vi "Endpoint Aliases Page.vi"(8 "error in (no error)":errorcluster, 11 "Node Ptr":T5 format="%.0x") -> (0 "error out":errorcluster)   [LabVIEW 2017, in "Routing and Faulting System Explorer.lvlib"]
uses:
  Routing and Faulting System Explorer.lvlib
  <vilib>/NI Veristand/Custom Device API/Custom Device Item Ref.ctl
  Alias.ctl
  Endpoint.ctl
  Shared/UI Common/Sort Button.ctl
  Shared/UI Common/Add Button.ctl
  Aliases Page Controls.ctl
  9b1be06d-3bcf-4b89-8ea1-6f7bb6167b61.vi
  Shared/UI Common/Set Control Value.vi
  <vilib>/NI Veristand/Custom Device API/Custom Device API.lvlib
  Shared/UI Common/UI Common.lvlib
  Scripting/Routing and Faulting Scripting.lvlib
panel:
  in  "Items to add":dbl=5.0
  in  "Add Alias":T1
  in  "Sort":T2
  out "Alias":string="Alias"
  out "Endpoint":string="Endpoint"
  in  "Aliases":T3[](array[typedef])
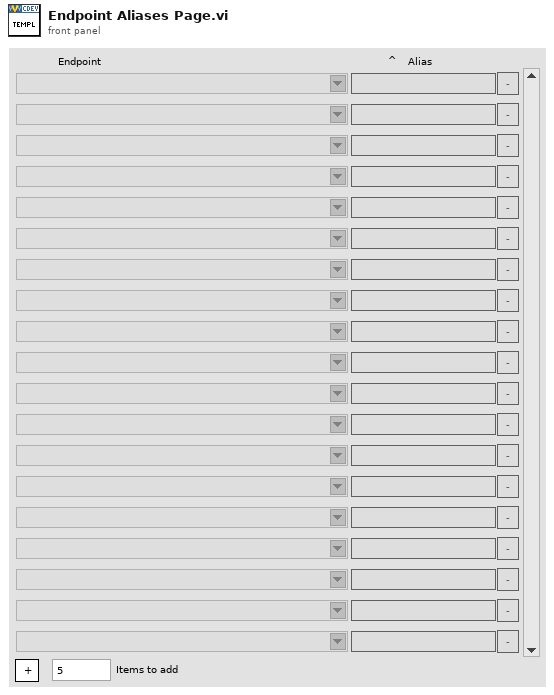
[diagram p1: front panel]
types:
  T1 = typedef "UI Common.lvlib/Add Button.ctl" = bool
  T2 = typedef "UI Common.lvlib/Sort Button.ctl" = bool
  T3 = typedef "Routing and Faulting System Explorer.lvlib/Alias.ctl" = cluster{"Endpoint":T4, "Alias":string, "Remove":bool}
  T4 = typedef "Routing and Faulting System Explorer.lvlib/Endpoint.ctl" = string
  T5 = typedef "Custom Device API.lvlib/Custom Device Item Ref.ctl" = u64
  T6 = typedef "Routing and Faulting System Explorer.lvlib/Aliases Page Controls.ctl" = cluster{"Aliases":refnum<vi>, "Endpoint":refnum<vi>, "Alias":refnum<vi>, "Sort":refnum<vi>}
  T7 = typedef "Custom Device API.lvlib/Custom Device Commands.ctl" = enum16{"Default", "Item renamed", "Shutdown", "Dynamic button pressed"}
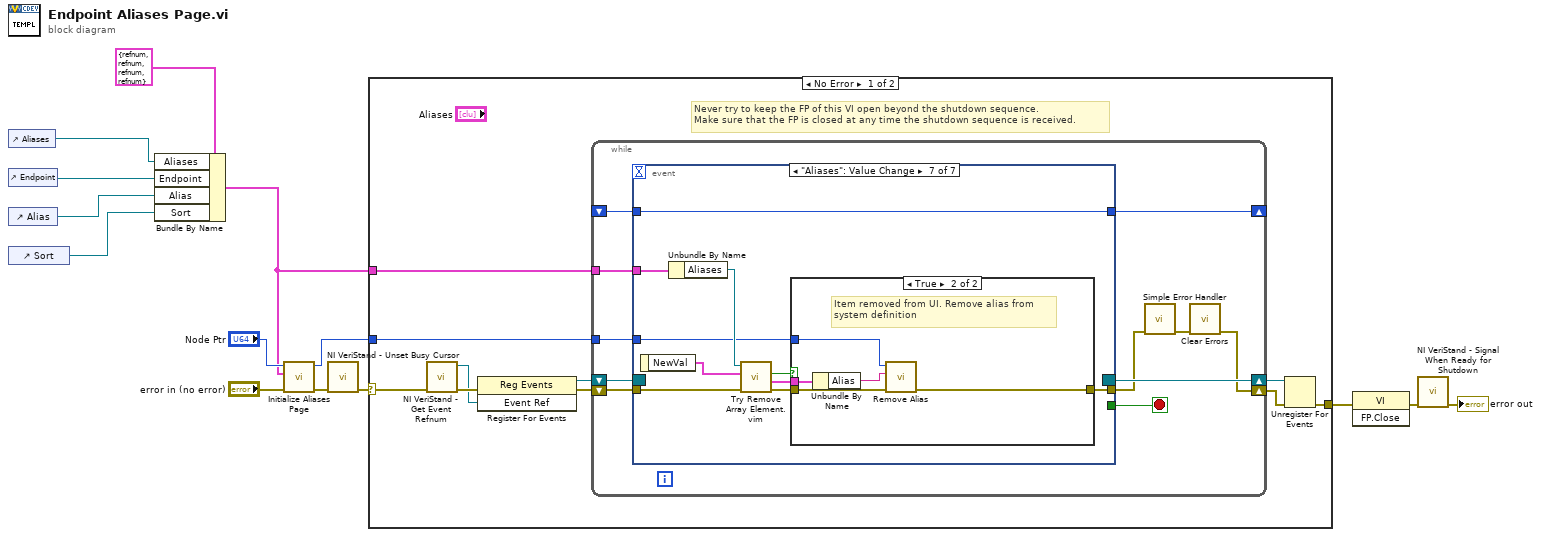
[diagram p0: block diagram]
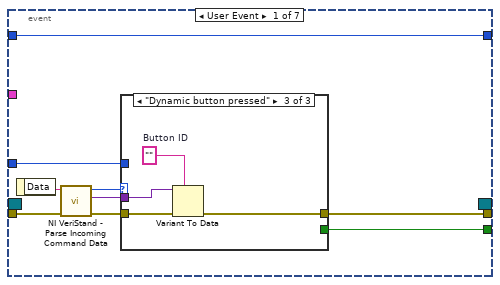
[diagram p2: hidden frame]
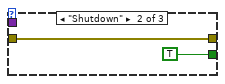
[diagram p4: hidden frame]
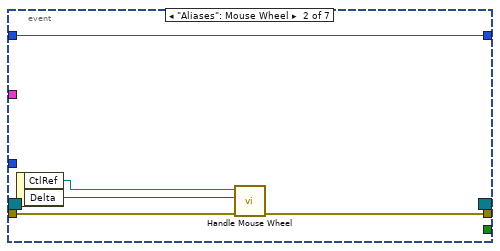
[diagram p5: hidden frame]
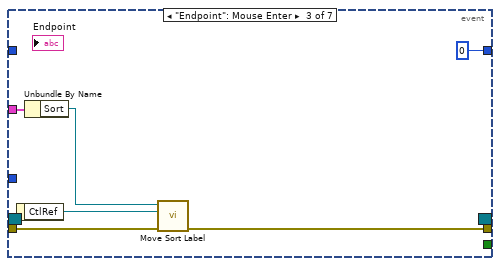
[diagram p6: hidden frame]
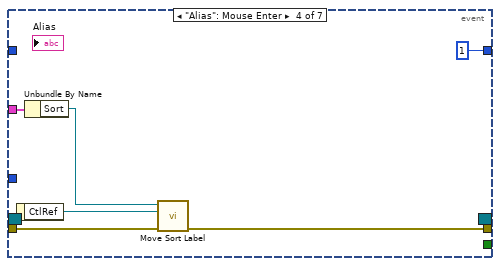
[diagram p7: hidden frame]
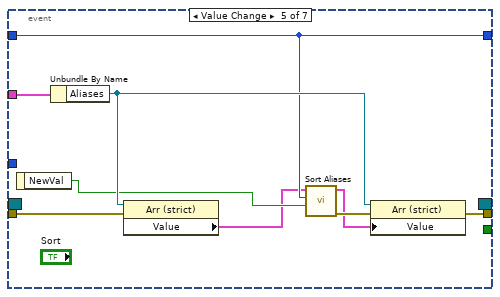
[diagram p8: hidden frame]
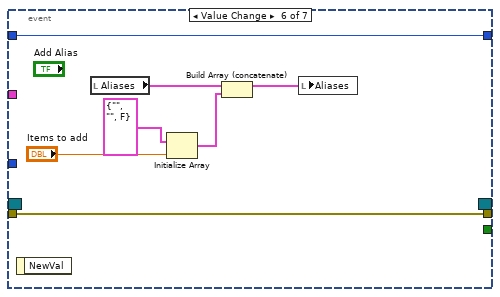
[diagram p9: hidden frame]
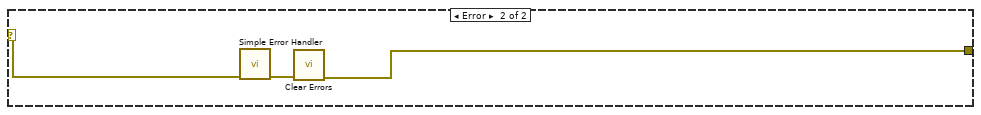
[diagram p11: hidden frame]
diagram:
  n1 = control-ref of="Aliases"() -> (w1:refnum<vi>)
  n2 = control-ref of="Endpoint"() -> (w8:refnum<vi>)
  n3 = control-ref of="Alias"() -> (w7:refnum<vi>)
  n4 = control-ref of="Sort"() -> (w6:refnum<vi>)
  n5 = Bundle By Name(cluster=T6 {"Aliases"=refnum, "Endpoint"=refnum, "Alias"=refnum, "Sort"=refnum} ("Aliases Page Controls"), "Aliases"=w1, "Endpoint"=w8, "Alias"=w7, "Sort"=w6) -> (w2:T6)
  n6 = call "Initialize Aliases Page.vi"("error in (no error)"="error in (no error)", "Aliases Page Controls"=w2, "Aliases Ref in"="Node Ptr") -> ("error out"=w5:errorcluster, "Aliases Ref out"=w9:T5)  [unwired: 7 in]
  n7 = call <vilib>:"NI VeriStand - Unset Busy Cursor.vi"("error in (no error)"=w5) -> ("error out"=w12:errorcluster)  [unwired: 10 out]
  n8 = case shown="No Error" w12 {
    selector: w12 -> [w19 w103]
    tunnel: [w22 w101] -> w14
    tunnel: w9 -> [w20 _]
    tunnel: w2 -> [w17 _]
    frame No Error {
      # "Never try to keep the FP of this VI open beyond the shutdown sequence.\nMake sure that the FP is closed at any time the shutdown sequence is received."
      n9 = call <vilib>:"NI VeriStand - Get Event Refnum.vi"("error in (no error)"=w19) -> ("error out"=w16:errorcluster, "Event Ref"=w15:refnum<user-event>)  [unwired: 9 out]
      n10 = register-events(error in=w16, w15) -> (reference out=w21:refnum<event-registration>, error out=w18:errorcluster)  [unwired: 1 in]
      n11 = while {
        tunnel: w20 -> [w31]
        shift-right: [w28] -> w23
        shift-left: w18 -> [w34]
        shift-right: [w35] -> w24
        shift-left: w21 -> [w33]
        shift-right: [w27] -> _
        shift-left: _ -> [w25]
        tunnel: w17 -> [w26]
        stop <- w32 stop-if-true
        n12 = event shown="[6] \"Aliases\": Value Change" {
          selector: w33 -> [_ _ _ _ _ _ _]
          dyn-events: [_ _ _ _ _ _ _] -> w35
          timeout: _ -> [_ _ _ _ _ _ _]
          tunnel: w34 -> [w44 w54 w62 w68 w77 w82 w93]
          tunnel: [w40 _ _ _ _ _ _] -> w32
          tunnel: [w39 w53 w61 w67 w74 w82 w87] -> w30
          tunnel: w31 -> [w38 _ _ _ _ _ w85]
          tunnel: [w36 w56 0 ("index of element") 1 ("index of element") w71 w84 w94] -> w27
          tunnel: w26 -> [_ _ w58 w64 w76 _ w91]
          tunnel: w25 -> [w36 w56 _ _ w71 w84 w94]
          event User Event {
            n13 = event-data() -> ("Data"=w43:string)  [unwired: 1 out]
            n14 = call <vilib>:"NI VeriStand - Parse Incoming Command Data.vi"("error in (no error)"=w44, "Incoming data"=w43) -> ("error out"=w42:errorcluster, "Outgoing data"=w37:variant, "Action"=w41:T7)  [unwired: 7 out]
            n15 = case shown="\"Dynamic button pressed\"" w41 {
              tunnel: w42 -> [w45 w46 w51]
              tunnel: [_ TRUE _] -> w40
              tunnel: [w45 w46 w48] -> w39
              tunnel: w38 -> [_ _ _]
              tunnel: w37 -> [_ _ w50]
              frame "Default", Default {
              }
              frame "Shutdown" {
              }
              frame "Dynamic button pressed" {
                w49 = ""  # Button ID
                n16 = Variant To Data(error in=w51, type=w49, Variant=w50) -> (error out=w48:errorcluster)  [unwired: 1 out]
              }
            }
          }
          event "Aliases": Mouse Wheel {
            n17 = event-data() -> ("CtlRef"=w55:refnum<vi>, "Delta"=w52:i32)  [unwired: 1 out]
            n18 = call "Handle Mouse Wheel.vi"("error in (no error)"=w54, "delta"=w52, "Array Refnum"=w55) -> ("error out"=w53:errorcluster)  [unwired: 7 in, 1 out]
          }
          event "Endpoint": Mouse Enter {
            n19 = event-data() -> ("CtlRef"=w60:refnum<vi>)  [unwired: 1 out]
            n20 = Unbundle By Name(w58) -> ("Sort"=w57:refnum<vi>)
            n21 = call "Move Sort Label.vi"("error in (no error)"=w62, "Target Label"=w60, "Sort"=w57) -> ("error out"=w61:errorcluster)  [unwired: 8 in]
          }
          event "Alias": Mouse Enter {
            n22 = event-data() -> ("CtlRef"=w66:refnum<vi>)  [unwired: 1 out]
            n23 = Unbundle By Name(w64) -> ("Sort"=w63:refnum<vi>)
            n24 = call "Move Sort Label.vi"("error in (no error)"=w68, "Target Label"=w66, "Sort"=w63) -> ("error out"=w67:errorcluster)  [unwired: 8 in]
          }
          event Value Change {
            n25 = event-data() -> ("NewVal"=w72:T2)  [unwired: 1 out]
            n26 = Unbundle By Name(w76) -> ("Aliases"=w73:refnum<vi>)
            n27 = property class="Arr (strict)"(reference=w73, error in=w77) -> ("Value"=w69:T3[])  [unwired: 2 out]
            n28 = call "Sort Aliases.vi"("Descending"=w72, "index"=w71, "Aliases"=w69) -> ("error out"=w75:errorcluster, "Sorted Aliases"=w70:T3[])  [unwired: 7 in]
            n29 = property class="Arr (strict)"(reference=w73, error in=w75, "Value"=w70) -> (error out=w74:errorcluster)  [unwired: 1 out]
          }
          event Value Change {
            n30 = event-data() -> ()  [unwired: 2 out]
            n31 = local read "Aliases"() -> (w80:T3[])
            n32 = Initialize Array(T3 {"Endpoint"="", "Alias"="", "Remove"=FALSE} ("Alias"), "Items to add") -> (w79:T3[])
            n33 = Build Array (concatenate)(w80, w79) -> (w78:T3[])
            n34 = local write "Aliases"(w78) -> ()
          }
          event "Aliases": Value Change {
            n35 = event-data() -> ("NewVal"=w92:T3[])  [unwired: 1 out]
            n36 = Unbundle By Name(w91) -> ("Aliases"=w90:refnum<vi>)
            n37 = call "Try Remove Array Element.vim"("error in (no error)"=w93, "Array"=w92, "Ctl Refnum"=w90) -> ("error out"=w88:errorcluster, "Removed Item"=w86:T3, "Removed?"=w89:bool)  [unwired: 5 in, 1 out]
            n38 = case shown="True" w89 {
              tunnel: w88 -> [w95 w99]
              tunnel: [w95 w98] -> w87
              tunnel: w86 -> [_ w100]
              tunnel: w85 -> [_ w96]
              frame False {
                # "No removal, something else happened.\nUpdate aliases accordingly."
              }
              frame True {
                # "Item removed from UI. Remove alias from\nsystem definition"
                n39 = Unbundle By Name(w100) -> ("Alias"=w97:string)
                n40 = call "Remove Alias.vi"("error in (no error)"=w99, "Alias"=w97, "Endpoint Aliases Ref in"=w96) -> ("error out"=w98:errorcluster)  [unwired: 7 in, 1 out]
              }
            }
          }
        }
        n41 = call <vilib>:"Simple Error Handler.vi"("error in (no error)"=w30) -> ("error out"=w29:errorcluster)  [unwired: 1 in, 7 out]
        n42 = call <vilib>:"Clear Errors.vi"("error in (no error)"=w29) -> ("error out"=w28:errorcluster)  [unwired: 1 in, 5 out]
      }
      n43 = Unregister For Events(event registration refnum=w24, error in=w23) -> (error out=w22:errorcluster)
    }
    frame Error {
      n44 = call <vilib>:"Simple Error Handler.vi"("error in (no error)"=w103) -> ("error out"=w102:errorcluster)  [unwired: 1 in, 7 out]
      n45 = call <vilib>:"Clear Errors.vi"("error in (no error)"=w102) -> ("error out"=w101:errorcluster)  [unwired: 1 in, 5 out]
    }
  }
  n46 = invoke class="VI" method="FP.Close"(error in=w14) -> (error out=w4:errorcluster)  [unwired: 2 in, 2 out]
  n47 = call <vilib>:"NI VeriStand - Signal When Ready for Shutdown.vi"("error in (no error)"=w4) -> ("error out"=→"error out":errorcluster)  [unwired: 10 out]
